vi "KNRm_image_recovery.vi"() -> ()   [LabVIEW 2019]
uses:
  <vilib>/nisyscfg/Network Settings Image.ctl
  <vilib>/nisyscfg/Set System Image (Folder).vi
  <vilib>/nisyscfg/nisyscfg.lvlib
panel:
  out "String":string
  out "fail":bool
  in  "Choose a Target then Run the VI":refnum<k21>
  out "display":i32(slide) caption="100%" scale=0.1..100.0
  out "error out":errorcluster
  # "OS6"
  # "Recovery Utility"
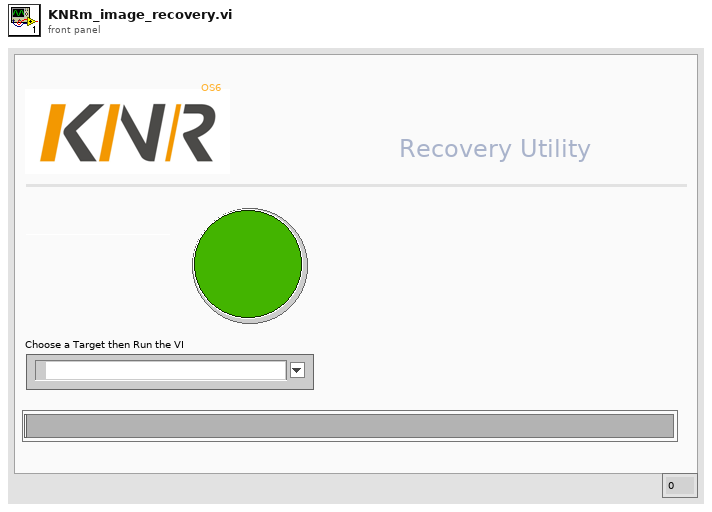
[diagram p1: front panel]
types:
  T1 = typedef "nisyscfg.lvlib/Network Settings Image.ctl" = u32
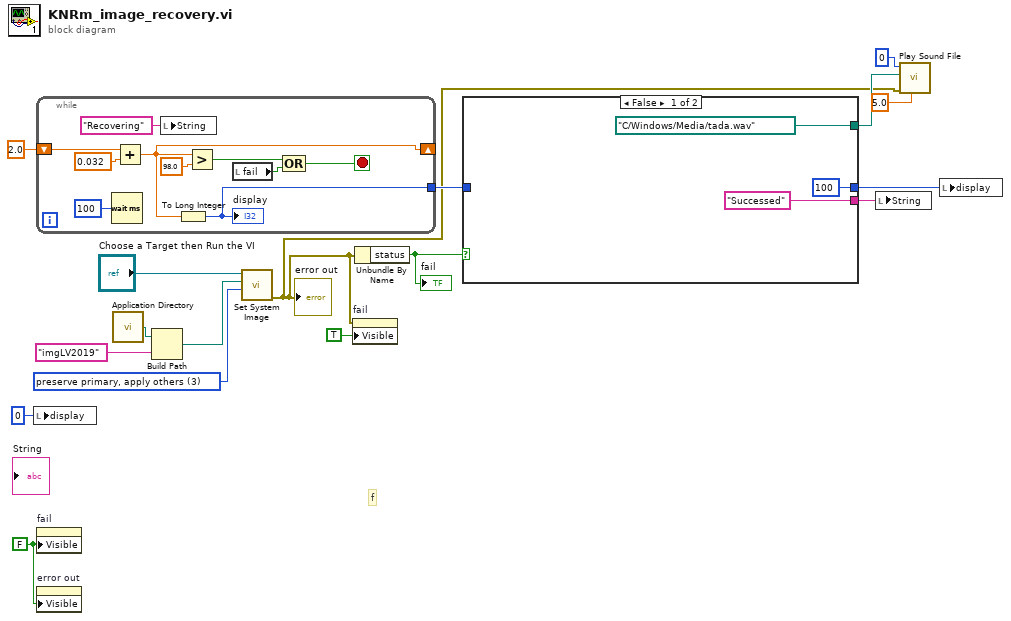
[diagram p0: block diagram]
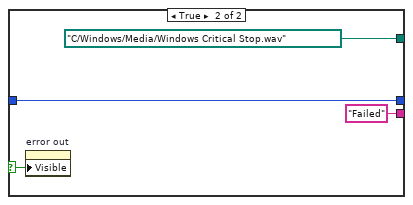
[diagram p2: hidden frame]
diagram:
  w3 = FALSE ("Visible")
  w15 = T1 3 items=["reset all network adapters", "preserve primary, reset others", "preserve all network adapters", "preserve primary, apply others", "apply primary, reset others", "apply primary, preserve others", "apply all network adapters"] ("Network Settings (preserve primary adapter, apply others)")
  # "f"
  n1 = local write "display"(0 ("display")) -> ()
  n2 = while {
    shift-right: [w20] -> _
    shift-left: 2.0 -> [w24]
    tunnel: [w19] -> w7
    stop <- w22 stop-if-true
    n3 = Wait (ms)(milliseconds to wait=u32 100) -> ()  [unwired: 1 out]
    n4 = Add(x=w24, y=0.032) -> (x+y=w20:dbl)
    n5 = local write "String"("Recovering" ("String")) -> ()
    n6 = To Long Integer(number=w20) -> (32bit integer=w19:i32)
    "display" <- w19
    n7 = Greater?(x=w20, y=98.0) -> (0:w26:bool)
    n8 = local read "fail"() -> (w21:bool)
    n9 = Compound Arithmetic op=OR(w26, w21) -> (w22:bool)
  }
  n10 = property on="fail" class="Bool (strict)"("Visible"=w3) -> ()  [unwired: 2 in, 2 out]
  n11 = property on="error out" class="Clust (strict)"("Visible"=w3) -> ()  [unwired: 2 in, 2 out]
  n12 = call <vilib>:"Application Directory.vi"() -> ("Application Directory"=w12:path)
  n13 = Build Path(base path=w12, name or relative path="imgLV2019") -> (appended path=w16:path)
  n14 = call-poly <vilib>:"Set System Image.vi"("Network Settings (preserve primary adapter, apply others)"=w15, "Source Folder"=w16, "Session in"="Choose a Target then Run the VI") -> ("error out"=w4:errorcluster)  [unwired: 7 in, 1 out]
  "error out" <- w4
  n15 = property on="fail" class="Bool (strict)"(error in=w4, "Visible"=TRUE) -> ()  [unwired: 1 in, 2 out]
  n16 = Unbundle By Name(w4) -> ("status"=w9:bool)
  "fail" <- w9
  n17 = case shown="False" w9 {
    selector: w9 -> [_ w32]
    tunnel: [100 ("display") w34] -> w8
    tunnel: w7 -> [_ w34]
    tunnel: [path "C:/Windows/Media/tada.wav" ("path") path "C:/Windows/Media/Windows Critical Stop.wav" ("path")] -> w6
    tunnel: ["Successed" ("String") "Failed" ("String")] -> w1
    frame False {
    }
    frame True {
      n18 = property on="error out" class="Clust (strict)"("Visible"=w32) -> ()  [unwired: 2 in, 2 out]
    }
  }
  n19 = local write "String"(w1) -> ()
  n20 = call <vilib>:"Play Sound File.vi"("timeout (sec)"=5.0, "error in (no error)"=w4, "path"=w6, "device ID"=u32 0) -> ()  [unwired: 6 in, 2 out]
  n21 = local write "display"(w8) -> ()
